vi "Create 256 Values Palette.vi"(5 "Image High Color":u32(colorbox)=16777216, 7 "Image Low Color":u32(colorbox)=16777216, 8 "Error In":errorcluster, 9 "Source Image Display Range":cluster{"Min Value":dbl, "Max Value":dbl}={"Min Value"=nan, "Max Value"=nan}, 10 "Interpolate?":bool, 11 "Palette Colors in":u32[](array[colorbox])) -> (0 "Error Out":errorcluster, 1 "Color Scale Marker Values":cluster{"Value":dbl, "Color":u32}[](array[cluster]), 2 "1D U32 array":u32[](array[colorbox]), 3 "1D Color value array":cluster{"Red":u8, "Green":u8, "Blue":u8}[](array[cluster]))   [LabVIEW 2021, in "Palette.lvlib"]
uses:
  Palette.lvlib
  <vilib>/vision/NI_Vision_Development_Module.lvlib
  Utilities/Utilities.lvlib
panel:
  out "Color Ramp":dbl(ramp)
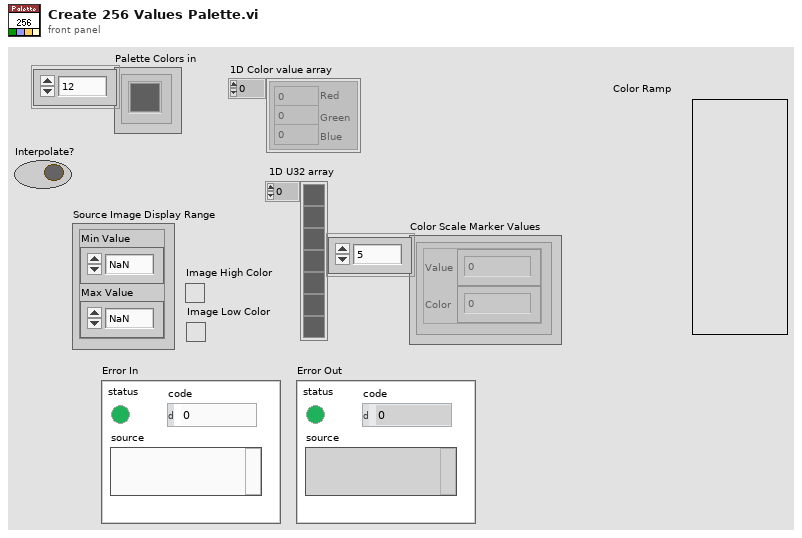
[diagram p1: front panel]
types:
  T1 = typedef "Utilities.lvlib/For Loop Iteration Type.ctl" = enum16{"default", "first", "last", "out of range"}
  T2 = cluster{"Red (or Hue) value":u8, "Green (or Sat) value":u8, "Blue (or Light or Val) value":u8}[]
  T3 = cluster{"Red (or Hue) value":u8, "Green (or Sat) value":u8, "Blue (or Light or Val) value":u8}
  T4 = cluster{"Numeric Control":dbl, "Numeric Control":u32}
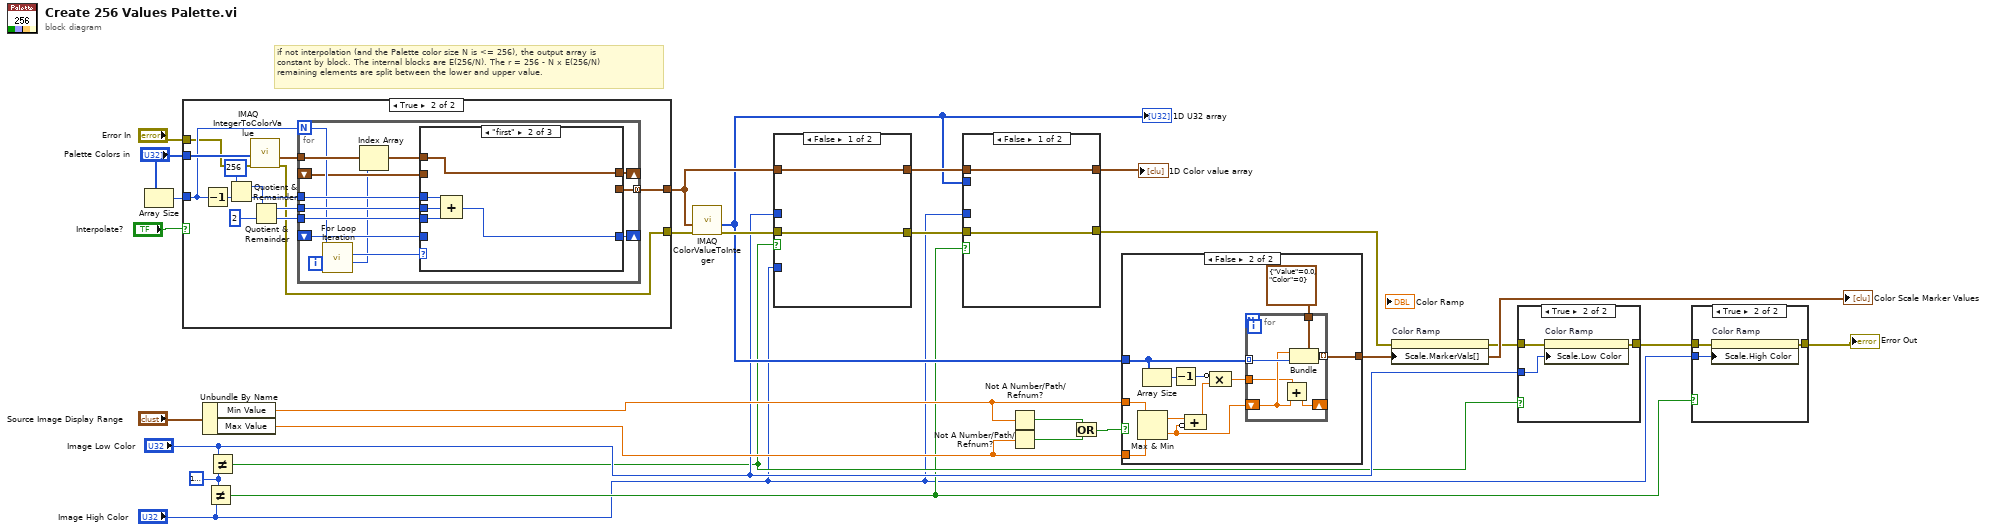
[diagram p0: block diagram]
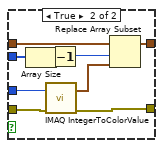
[diagram p4: hidden frame]
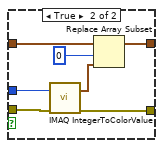
[diagram p5: hidden frame]
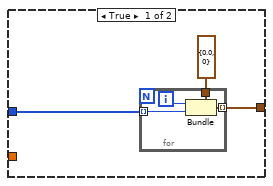
[diagram p6: hidden frame]
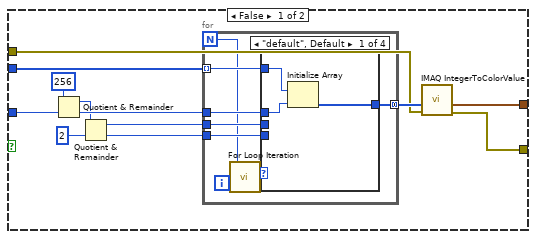
[diagram p7: hidden frame]
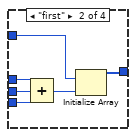
[diagram p8: hidden frame]
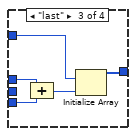
[diagram p9: hidden frame]
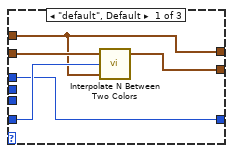
[diagram p11: hidden frame]
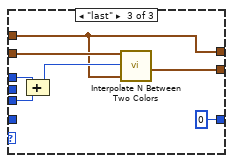
[diagram p12: hidden frame]
diagram:
  w13 = u32 16777216 ("Image Low Color")
  # "if not interpolation (and the Palette color size N is <= 256), the output array is\nconstant by block. The internal blocks are E(256/N). The r = 256 - N x E(256/N)\nremaining elements are split between the lower and upper value."
  n1 = Array Size(array="Palette Colors in") -> (size(s)=w26:i32)
  n2 = case shown="True" "Interpolate?" {
    tunnel: w26 -> [w39 w65]
    tunnel: "Palette Colors in" -> [w34 w68]
    tunnel: [w30 w66] -> w17
    tunnel: "Error In" -> [w29 w63]
    tunnel: [w28 w62] -> w15
    frame False {
      n3 = Quotient & Remainder(x=256, y=w39) -> (x-y*floor(x/y)=w37:i32, floor(x/y)=w38:i32)
      n4 = Quotient & Remainder(x=w37, y=2) -> (x-y*floor(x/y)=w35:i32, floor(x/y)=w33:i32)
      n5 = for {
        N -> [w40]
        tunnel: w38 -> [w45]
        tunnel: w33 -> [w47]
        tunnel: w35 -> [w46]
        tunnel: w34 -> [w43] mode=indexing
        tunnel: [w44] -> w31 mode=concatenating
        i -> [w42]
        n6 = call "For Loop Iteration.vi"("i"=w42, "N"=w40) -> ("Iteration"=w41:T1)  [unwired: 8 in, 1 out]
        n7 = case shown="\"default\", Default" w41 {
          tunnel: w47 -> [_ w56 w61 _]
          tunnel: w46 -> [_ w55 _ _]
          tunnel: w45 -> [w50 w54 w60 _]
          tunnel: w43 -> [w49 w52 w58 _]
          tunnel: [w48 w51 w57 _] -> w44
          frame "default", Default {
            n8 = Initialize Array(w49, w50) -> (w48:u32[])
          }
          frame "first" {
            n9 = Compound Arithmetic op=ADD(w54, w55, w56) -> (w53:i32)
            n10 = Initialize Array(w52, w53) -> (w51:u32[])
          }
          frame "last" {
            n11 = Compound Arithmetic op=ADD(w60, w61) -> (w59:i32)
            n12 = Initialize Array(w58, w59) -> (w57:u32[])
          }
          frame "out of range" {
          }
        }
      }
      n13 = call "IMAQ IntegerToColorValue"("error in (no error)"=w29, "1D U32 array"=w31) -> ("1D Color value array"=w30:T2, "error out"=w28:errorcluster)  [unwired: 3 in, 2 out]
    }
    frame True {
      n14 = Decrement(x=w65) -> (x-1=w64:i32)
      n15 = Quotient & Remainder(x=256, y=w64) -> (x-y*floor(x/y)=w73:i32, floor(x/y)=w74:i32)
      n16 = call "IMAQ IntegerToColorValue"("error in (no error)"=w63, "1D U32 array"=w68) -> ("1D Color value array"=w67:T2, "error out"=w62:errorcluster)  [unwired: 3 in, 2 out]
      n17 = Quotient & Remainder(x=w73, y=2) -> (x-y*floor(x/y)=w71:i32, floor(x/y)=w70:i32)
      n18 = for {
        N: w65 -> [w84]
        tunnel: w74 -> [w86]
        tunnel: w70 -> [w88]
        tunnel: w71 -> [w87]
        tunnel: w67 -> [w85]
        shift-right: [w81] -> _
        shift-left: _ -> [w79]
        shift-right: [w80] -> _
        shift-left: _ -> [w78]
        tunnel: [w77] -> w66 mode=concatenating
        i -> [w83]
        n19 = call "For Loop Iteration.vi"("i"=w83, "N"=w84) -> ("i (dup)"=w75:i32, "Iteration"=w82:T1)  [unwired: 8 in]
        n20 = Index Array(array=w85, index=w75) -> (element=w76:T3)
        n21 = case shown="\"first\"" w82 {
          tunnel: w88 -> [_ w98 w105]
          tunnel: w87 -> [_ w97 _]
          tunnel: w86 -> [w91 w96 w104]
          tunnel: w76 -> [w89 w95 w100]
          tunnel: [w89 w95 w100] -> w81
          tunnel: [w91 w94 0] -> w80
          tunnel: w79 -> [w90 _ w101]
          tunnel: w78 -> [w92 _ _]
          tunnel: [w93 _ w103] -> w77
          frame "default", Default {
            n22 = call "Interpolate N Between Two Colors.vi"("Starting Color Value"=w90, "# Elements"=w92, "Ending Color Value"=w89) -> ("Color Array"=w93:T2)  [unwired: 6 in]
          }
          frame "first" {
            n23 = Compound Arithmetic op=ADD(w96, w97, w98) -> (w94:i32)
          }
          frame "last" {
            n24 = Compound Arithmetic op=ADD(w104, w105) -> (w102:i32)
            n25 = call "Interpolate N Between Two Colors.vi"("Starting Color Value"=w101, "# Elements"=w102, "Ending Color Value"=w100) -> ("Color Array"=w103:T2)  [unwired: 6 in]
          }
        }
      }
    }
  }
  n26 = Unbundle By Name("Source Image Display Range") -> ("Min Value"=w21:dbl, "Max Value"=w20:dbl)
  n27 = Not Equal?(x=w13, y="Image High Color") -> (x != y?=w4:bool)
  n28 = Not Equal?(x="Image Low Color", y=w13) -> (x != y?=w6:bool)
  n29 = call "IMAQ ColorValueToInteger"("error in (no error)"=w15, "1D Color value array"=w17) -> ("1D U32 array"=w10:u32[], "error out"=w14:errorcluster)  [unwired: 3 in, 2 out]
  "1D U32 array" <- w10
  n30 = case shown="False" w6 {
    tunnel: w17 -> [w107 w114]
    tunnel: [w107 w111] -> w12
    tunnel: w14 -> [w106 w110]
    tunnel: "Image Low Color" -> [_ w109]
    tunnel: "Image High Color" -> [_ _]
    tunnel: [w106 w108] -> w9
    frame False {
    }
    frame True {
      n31 = call "IMAQ IntegerToColorValue"("error in (no error)"=w110, "U32 value"=w109) -> ("error out"=w108:errorcluster, "Color Value"=w112:T3)  [unwired: 3 in, 2 out]
      n32 = Replace Array Subset(array=w114, new element=w112, index=0) -> (w111:T2)
    }
  }
  n33 = case shown="False" w4 {
    tunnel: w12 -> [w116 w124]
    tunnel: [w116 w122] -> w11
    tunnel: w10 -> [_ w121]
    tunnel: w9 -> [w115 w120]
    tunnel: "Image High Color" -> [_ w119]
    tunnel: [w115 w117] -> w1
    frame False {
    }
    frame True {
      n34 = Array Size(array=w121) -> (size(s)=w125:i32)
      n35 = call "IMAQ IntegerToColorValue"("error in (no error)"=w120, "U32 value"=w119) -> ("error out"=w117:errorcluster, "Color Value"=w123:T3)  [unwired: 3 in, 2 out]
      n36 = Decrement(x=w125) -> (x-1=w118:i32)
      n37 = Replace Array Subset(array=w124, new element=w123, index=w118) -> (w122:T2)
    }
  }
  "1D Color value array" <- w11
  n38 = Not A Number/Path/Refnum?(number/path/refnum=w21) -> (NaN/Path/Refnum?=w24:bool)
  n39 = Not A Number/Path/Refnum?(number/path/refnum=w20) -> (NaN/Path/Refnum?=w23:bool)
  n40 = Or(x=w24, y=w23) -> (x .or. y?=w18:bool)
  n41 = case shown="False" w18 {
    tunnel: w10 -> [w128 w139]
    tunnel: [w127 w143] -> w19
    tunnel: w20 -> [_ w140]
    tunnel: w21 -> [_ w141]
    frame True {
      n42 = for {
        tunnel: w128 -> [w131] mode=indexing
        tunnel: [w130] -> w127 mode=indexing
        tunnel: T4 {"Numeric Control"=0.0, "Numeric Control"=0} ("Scale.Marker Values[]") -> [w129]
        i -> [w132]
        n43 = Bundle(cluster=w129, "Numeric Control"=w132, "Numeric Control"=w131) -> (w130:T4)
      }
    }
    frame False {
      n44 = Max & Min(x=w141, y=w140) -> (max(x,y)=w138:dbl, min(x,y)=w137:dbl)
      n45 = Array Size(array=w139) -> (size(s)=w134:i32)
      n46 = Decrement(x=w134) -> (x-1=w133:i32)
      n47 = Compound Arithmetic op=ADD(w138, invert w137) -> (w136:dbl)
      n48 = Compound Arithmetic op=MULTIPLY(invert w133, w136) -> (w135:dbl)
      n49 = for {
        tunnel: w139 -> [w149] mode=indexing
        tunnel: [w148] -> w143 mode=indexing
        tunnel: cluster{"Value":dbl, "Color":u32} {"Value"=0.0, "Color"=0} ("Scale.Marker Values[]") -> [w147]
        shift-right: [w144] -> _
        shift-left: w137 -> [w146]
        tunnel: w135 -> [w145]
        n50 = Add(x=w145, y=w146) -> (x+y=w144:dbl)
        n51 = Bundle(cluster=w147, "Value"=w146, "Color"=w149) -> (w148:cluster{"Value":dbl, "Color":u32})
      }
    }
  }
  "Color Scale Marker Values" <- w19
  n52 = property on="Color Ramp" class="ColRmp (strict)"(error in=w1, "Scale.MarkerVals[]"=w19) -> (error out=w8:errorcluster)  [unwired: 1 in, 1 out]
  n53 = case shown="True" w6 {
    tunnel: w8 -> [w150 w153]
    tunnel: "Image Low Color" -> [_ w152]
    tunnel: [w150 w151] -> w5
    frame False {
    }
    frame True {
      n54 = property on="Color Ramp" class="ColRmp (strict)"(error in=w153, "Scale.Low Color"=w152) -> (error out=w151:errorcluster)  [unwired: 1 in, 1 out]
    }
  }
  n55 = case shown="True" w4 {
    tunnel: w5 -> [w154 w157]
    tunnel: "Image High Color" -> [_ w156]
    tunnel: [w154 w155] -> w2
    frame False {
    }
    frame True {
      n56 = property on="Color Ramp" class="ColRmp (strict)"(error in=w157, "Scale.High Color"=w156) -> (error out=w155:errorcluster)  [unwired: 1 in, 1 out]
    }
  }
  "Error Out" <- w2
